vi "Untitled 1.vi"() -> ()   [LabVIEW 2017]
uses:
  <vilib>/Analysis/6fits.llb/1D B-Spline Fit.vi
  <vilib>/Analysis/NI_AALPro.lvlib
panel:
  out "error":i32
  in  "# of control points":i32=10
  out "1D B-Spline Fit on Arbitrary Curve":T1(graph)
  in  "parameter selection":u16(ring)=2 items=["equally spaced", "chord length", "centripetal"]
  out "Best BSpline Fit X":dbl[](array[numeric])
  out "Best BSpline Fit Y":dbl[](array[numeric])
  in  "Weight":dbl[](array[numeric])
  in  "X":dbl[](array[numeric])
  in  "Y":dbl[](array[numeric])
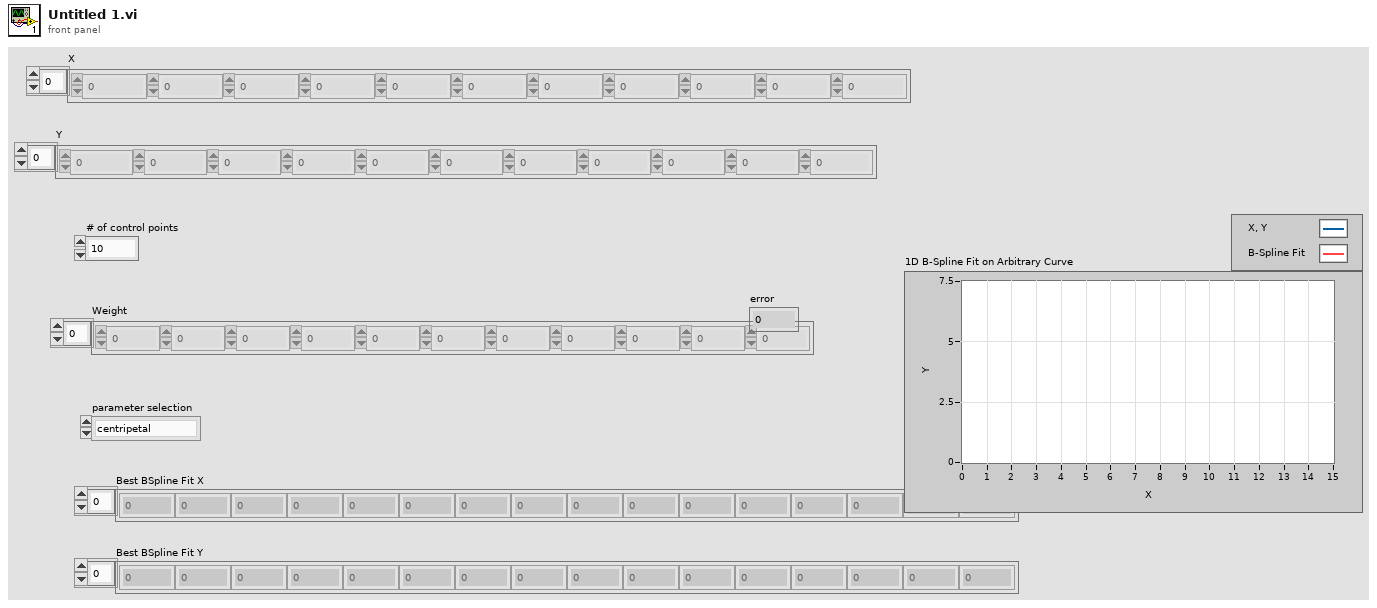
[diagram p1: front panel]
types:
  T1 = cluster{"Best BSpline Fit X":dbl[], "Best BSpline Fit Y":dbl[]}[]
  T2 = cluster{"Best BSpline Fit X":dbl[], "Best BSpline Fit Y":dbl[]}
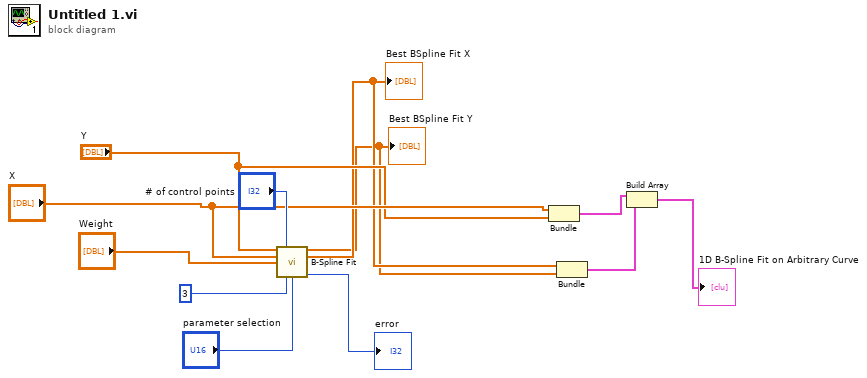
[diagram p0: block diagram]
diagram:
  n1 = call-poly <vilib>:"B-Spline Fit.vi"("Y"="Y", "# of control points"="# of control points", "X"="X", "Weight"="Weight", "degree"=3, "parameter selection"="parameter selection") -> ("Best BSpline Fit Y"=w3:dbl[], "Best BSpline Fit X"=w4:dbl[], "error"=→"error":i32)  [unwired: 6 in, 1 out]
  "Best BSpline Fit Y" <- w3
  "Best BSpline Fit X" <- w4
  n2 = Bundle("X"="X", "Y"="Y") -> (w6:cluster{"X":dbl[], "Y":dbl[]})  [unwired: 1 out]
  n3 = Bundle("Best BSpline Fit X"=w4, "Best BSpline Fit Y"=w3) -> (w2:T2)  [unwired: 1 out]
  n4 = Build Array(w6, w2) -> (→"1D B-Spline Fit on Arbitrary Curve":T1)
